vi "Check Parent Folder Selection.vi"(0 "Tree reference in":refnum<vi>, 5 "Child Tag":string, 11 "error in":errorcluster) -> (4 "Tree reference out":refnum<vi>, 15 "error out":errorcluster)   [LabVIEW 2021, in "Converter.lvlib"]
uses:
  Converter.lvlib
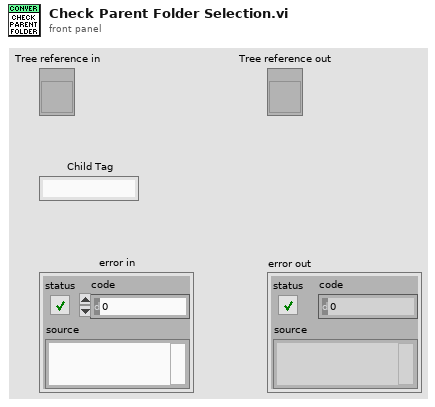
[diagram p1: front panel]
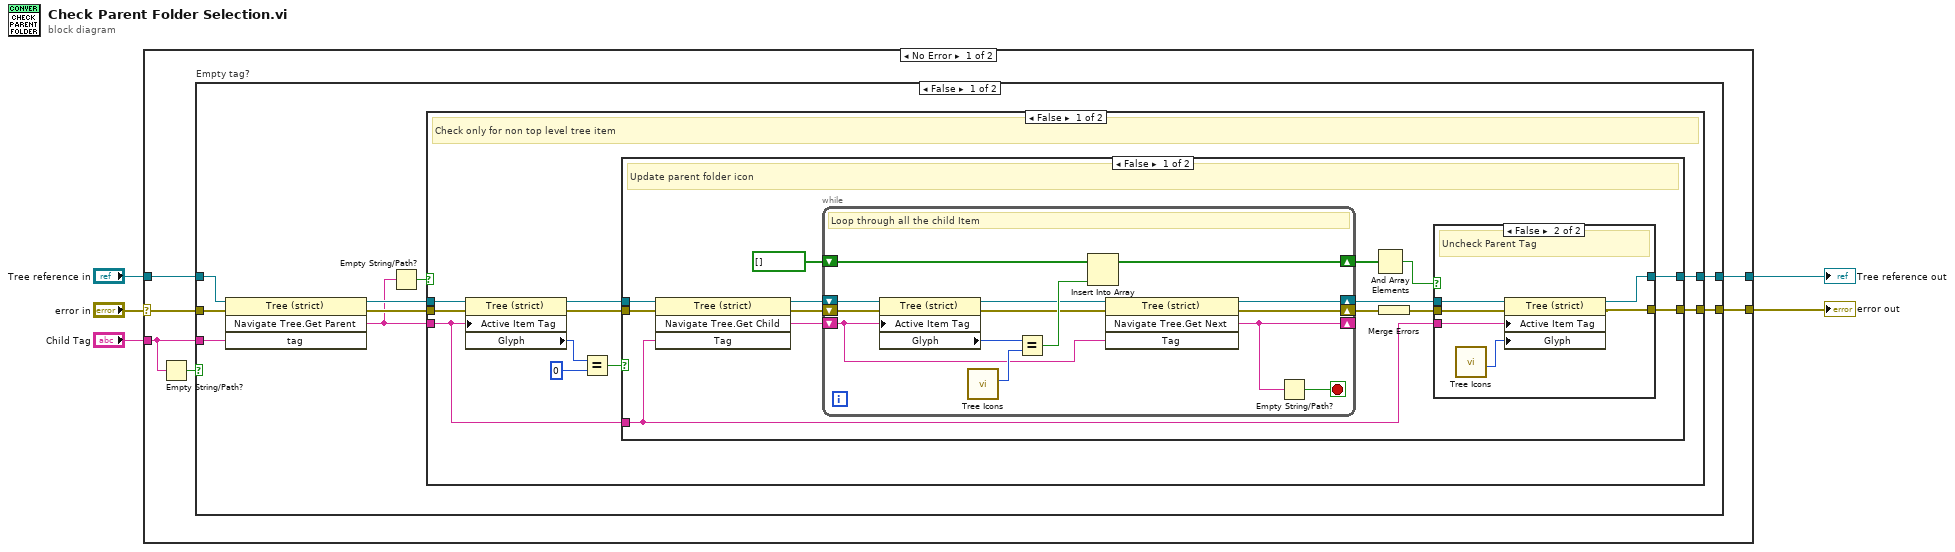
[diagram p0: block diagram]
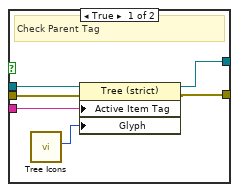
[diagram p2: hidden frame]
diagram:
  n1 = case shown="No Error" "error in" {
    selector: "error in" -> [w11 w78]
    tunnel: "Child Tag" -> [w7 _]
    tunnel: "Tree reference in" -> [w10 w77]
    tunnel: [w9 w78] -> w2
    tunnel: [w8 w77] -> w1
    frame No Error {
      n2 = Empty String/Path?(string/path=w7) -> (empty?=w6:bool)
      n3 = case "Empty tag?" shown="False" w6 {
        tunnel: w7 -> [w20 _]
        tunnel: w11 -> [w19 w75]
        tunnel: w10 -> [w16 w76]
        tunnel: [w13 w75] -> w9
        tunnel: [w12 w76] -> w8
        frame False {
          n4 = invoke class="Tree (strict)" method="Navigate Tree.Get Parent"(reference=w16, error in=w19, "tag"=w20) -> (reference out=w18:refnum<vi>, error out=w17:errorcluster, "Navigate Tree:Get Parent"=w14:string)  [unwired: 1 in, 1 out]
          n5 = Empty String/Path?(string/path=w14) -> (empty?=w15:bool)
          n6 = case shown="False" w15 {
            tunnel: w18 -> [w26 w73]
            tunnel: w14 -> [w21 _]
            tunnel: w17 -> [w27 w74]
            tunnel: [w30 w74] -> w13
            tunnel: [w29 w73] -> w12
            frame False {
              # "Check only for non top level tree item"
              n7 = property class="Tree (strict)"(reference=w26, error in=w27, "Active Item Tag"=w21) -> (reference out=w22:refnum<vi>, error out=w28:errorcluster, "Glyph"=w25:i32)
              n8 = Equal?(x=w25, y=0) -> (x = y?=w23:bool)
              n9 = case shown="False" w23 {
                tunnel: w22 -> [w44 w71]
                tunnel: w28 -> [w43 w72]
                tunnel: w21 -> [w35 _]
                tunnel: [w34 w72] -> w30
                tunnel: [w31 w71] -> w29
                frame False {
                  # "Update parent folder icon"
                  n10 = invoke class="Tree (strict)" method="Navigate Tree.Get Child"(reference=w44, error in=w43, "Tag"=w35) -> (reference out=w40:refnum<vi>, error out=w41:errorcluster, "Navigate Tree:Get Child"=w42:string)  [unwired: 1 in, 1 out]
                  n11 = while {
                    shift-right: [w46] -> _
                    shift-left: w42 -> [w48]
                    shift-right: [w52] -> w32
                    shift-left: w40 -> [w57]
                    shift-right: [w47] -> w37
                    shift-left: bool[] [] -> [w54]
                    shift-right: [w50] -> w38
                    shift-left: w41 -> [w58]
                    stop <- w45 stop-if-true
                    # "Loop through all the child Item"
                    n12 = property class="Tree (strict)"(reference=w57, error in=w58, "Active Item Tag"=w48) -> (reference out=w49:refnum<vi>, error out=w51:errorcluster, "Glyph"=w55:i32)
                    n13 = call "Tree Icons.vi"() -> ("Selected"=w56:i32)  [unwired: 6 in, 1 out]
                    n14 = Equal?(x=w55, y=w56) -> (x = y?=w53:bool)
                    n15 = Insert Into Array(array=w54, new element=w53) -> (w47:bool[])  [unwired: 1 in]
                    n16 = invoke class="Tree (strict)" method="Navigate Tree.Get Next"(reference=w49, error in=w51, "Tag"=w48) -> (reference out=w52:refnum<vi>, error out=w50:errorcluster, "Navigate Tree:Get Next Item"=w46:string)  [unwired: 1 in, 1 out]
                    n17 = Empty String/Path?(string/path=w46) -> (empty?=w45:bool)
                  }
                  n18 = And Array Elements(Boolean array=w37) -> (logical AND=w33:bool)
                  n19 = Merge Errors(w38) -> (w36:errorcluster)
                  n20 = case shown="False" w33 {
                    tunnel: w36 -> [w64 w70]
                    tunnel: w35 -> [w63 w69]
                    tunnel: [w62 w68] -> w34
                    tunnel: w32 -> [w60 w66]
                    tunnel: [w59 w65] -> w31
                    frame True {
                      # "Check Parent Tag"
                      n21 = call "Tree Icons.vi"() -> ("Selected"=w61:i32)  [unwired: 6 in, 1 out]
                      n22 = property class="Tree (strict)"(reference=w60, error in=w64, "Active Item Tag"=w63, "Glyph"=w61) -> (reference out=w59:refnum<vi>, error out=w62:errorcluster)
                    }
                    frame False {
                      # "Uncheck Parent Tag"
                      n23 = call "Tree Icons.vi"() -> ("Not Selected"=w67:i32)  [unwired: 6 in, 1 out]
                      n24 = property class="Tree (strict)"(reference=w66, error in=w70, "Active Item Tag"=w69, "Glyph"=w67) -> (reference out=w65:refnum<vi>, error out=w68:errorcluster)
                    }
                  }
                }
                frame True {
                }
              }
            }
            frame True {
              # "Skip if top level tree item"
            }
          }
        }
        frame True {
        }
      }
    }
    frame Error {
    }
  }
  "error out" <- w2
  "Tree reference out" <- w1
